vi "Initialize.vi"(8 "error in (no error)":errorcluster, 9 "Reset (True)":bool=TRUE, 10 "ID Query (True)":bool=TRUE, 11 "VISA resource name":refnum<visa-resource-name>) -> (0 "error out":errorcluster, 2 "idn string":string, 3 "VISA resource name out":refnum<visa-resource-name>, 5 "Model":u8(ring) items=["T3AWG3252", "T3AWG3352", "T3AWG3254", "T3AWG3354", "T3AWG3258", "T3AWG3358", "AWG4012", "AWG4014", "AWG4018", "Model675_2C", "Model675_4C", "Model675_8C", "Not valid"], 6 "Number of Markers Out":u8(ring) items=["1 Marker Out ", "2 Marker Out", "4 Marker Out"], 7 "Number of Channels Out":u8(ring) items=["2 Channels", "4 Channels", "8 Channels"])   [LabVIEW 2020, in "Active Technologies AWG3000.lvlib"]
doc: "Establishes communication with the instrument and optionally performs an instrument identification query and/or an instrument reset. It also places the instrument in a default state needed for other instrument driver operations. Therefore, call this VI before calling other instrument driver VIs for this instrument. Generally, you need to call the <B>Initialize VI</B> only once at the beginning of an application."
uses:
  Active Technologies AWG3000.lvlib
panel:
  in  "Timeout Value":u32=300000
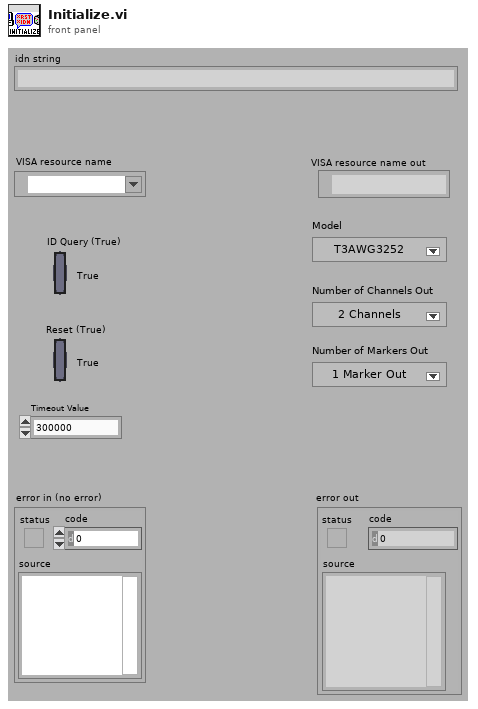
[diagram p1: front panel]
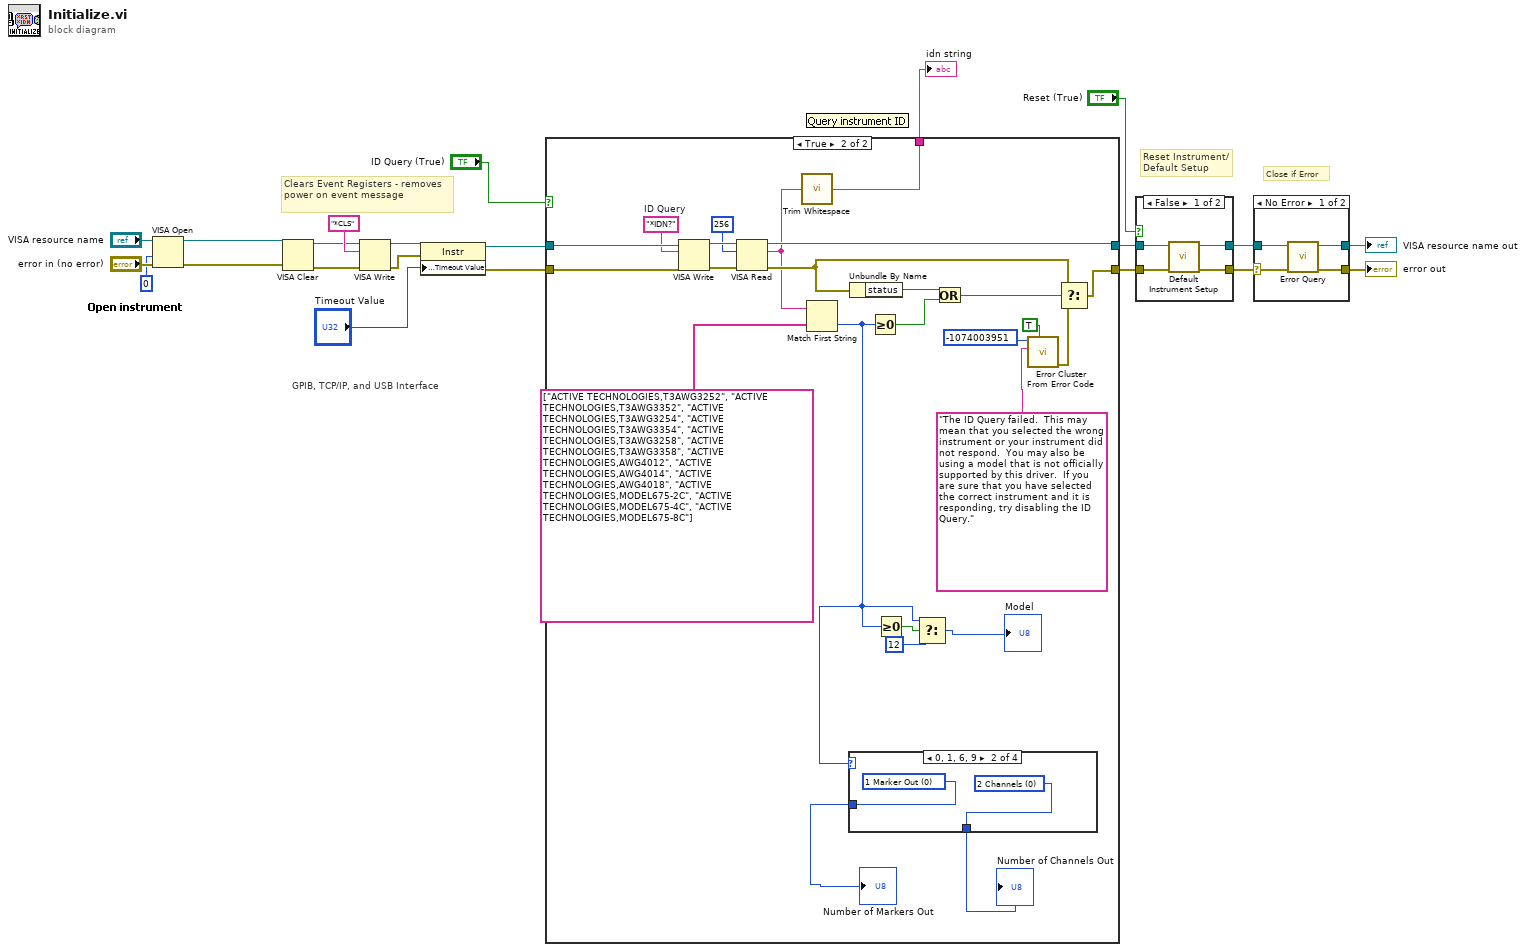
[diagram p0: block diagram]
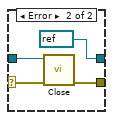
[diagram p2: hidden frame]
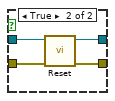
[diagram p3: hidden frame]
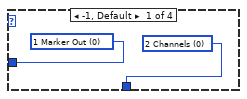
[diagram p5: hidden frame]
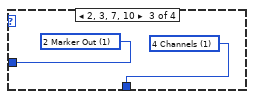
[diagram p6: hidden frame]
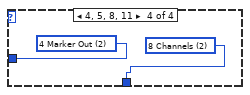
[diagram p7: hidden frame]
diagram:
  # "Clears Event Registers - removes power on event message"
  # "GPIB, TCP/IP, and USB Interface"
  # "Close if Error"
  # "Reset Instrument/\nDefault Setup"
  n1 = VISA Open(access mode=u32 0, error in (no error)="error in (no error)", VISA resource name="VISA resource name") -> (VISA resource name=w17:refnum<visa-resource-name>, error out=w16:errorcluster)  [unwired: 2 in]
  n2 = VISA Clear(VISA resource name=w17, error in (no error)=w16) -> (VISA resource name out=w5:refnum<visa-resource-name>, error out=w4:errorcluster)
  n3 = VISA Write(VISA resource name=w5, write buffer="*CLS", error in (no error)=w4) -> (VISA resource name out=w3:refnum<visa-resource-name>, error out=w2:errorcluster)  [unwired: 1 out]
  n4 = property class="Instr"(reference=w3, error in=w2, "General Settings:Timeout Value"="Timeout Value") -> (reference out=w9:refnum<visa-resource-name>, error out=w8:errorcluster)
  n5 = case shown="True" "ID Query (True)" {
    tunnel: [w23 w38] -> w10
    tunnel: [w24 w47] -> w11
    tunnel: w9 -> [w24 w48]
    tunnel: w8 -> [w23 w49]
    tunnel: [_ w25] -> w1
    frame False {
    }
    frame True {
      w43 = "*IDN?"  # ID Query
      n6 = VISA Write(VISA resource name=w48, write buffer=w43, error in (no error)=w49) -> (VISA resource name out=w46:refnum<visa-resource-name>, error out=w45:errorcluster)  [unwired: 1 out]
      n7 = VISA Read(VISA resource name=w46, byte count=u32 256, error in (no error)=w45) -> (VISA resource name out=w47:refnum<visa-resource-name>, read buffer=w26:string, error out=w42:errorcluster)  [unwired: 1 out]
      n8 = call <vilib>:"Trim Whitespace.vi"("string"=w26) -> ("trimmed string"=w25:string)  [unwired: 1 in]
      n9 = Match First String(2:string[] ["ACTIVE TECHNOLOGIES,T3AWG3252", "ACTIVE TECHNOLOGIES,T3AWG3352", "ACTIVE TECHNOLOGIES,T3AWG3254", "ACTIVE TECHNOLOGIES,T3AWG3354", "ACTIVE TECHNOLOGIES,T3AWG3258", "ACTIVE TECHNOLOGIES,T3AWG3358", "ACTIVE TECHNOLOGIES,AWG4012", "ACTIVE TECHNOLOGIES,AWG4014", "ACTIVE TECHNOLOGIES,AWG4018", "ACTIVE TECHNOLOGIES,MODEL675-2C", "ACTIVE TECHNOLOGIES,MODEL675-4C", "ACTIVE TECHNOLOGIES,MODEL675-8C"] ("reversed array"), 3:w26) -> (0:w30:i32)  [unwired: 1 out]
      n10 = case shown="0, 1, 6, 9" w30 {
        tunnel: [w51 w53 w55 w57] -> w33
        tunnel: [w50 w52 w54 w56] -> w32
        frame -1, Default {
          w50 = u8 0 items=["2 Channels", "4 Channels", "8 Channels"] ("Number of Channel Out")
          w51 = u8 0 items=["1 Marker Out ", "2 Marker Out", "4 Marker Out"] ("Number of Marker Out")
        }
        frame 0, 1, 6, 9 {
          w52 = u8 0 items=["2 Channels", "4 Channels", "8 Channels"] ("Number of Channel Out")
          w53 = u8 0 items=["1 Marker Out ", "2 Marker Out", "4 Marker Out"] ("Number of Marker Out")
        }
        frame 2, 3, 7, 10 {
          w54 = u8 1 items=["2 Channels", "4 Channels", "8 Channels"] ("Number of Channel Out")
          w55 = u8 1 items=["1 Marker Out ", "2 Marker Out", "4 Marker Out"] ("Number of Marker Out")
        }
        frame 4, 5, 8, 11 {
          w56 = u8 2 items=["2 Channels", "4 Channels", "8 Channels"] ("Number of Channel Out")
          w57 = u8 2 items=["1 Marker Out ", "2 Marker Out", "4 Marker Out"] ("Number of Marker Out")
        }
      }
      "Number of Markers Out" <- w33
      "Number of Channels Out" <- w32
      n11 = Unbundle By Name(w42) -> ("status"=w41:bool)
      n12 = Greater Or Equal To 0?(x=w30) -> (x >= 0?=w40:bool)
      n13 = Greater Or Equal To 0?(x=w30) -> (x >= 0?=w31:bool)
      n14 = Select(t=w30, s=w31, f=12) -> (s? t:f=→"Model":i32)
      n15 = Or(x=w41, y=w40) -> (x .or. y?=w39:bool)
      n16 = call <vilib>:"Error Cluster From Error Code.vi"("show call chain? (False)"=TRUE, "error message (\"\")"="The ID Query failed.  This may mean that you selected the wrong instrument or your instrument did not respond.  You may also be using a model that is not officially supported by this driver.  If you are sure that you have selected the correct instrument and it is responding, try disabling the ID Query." ("Source (VI Name)"), "error code (0)"=-1074003951 ("Code")) -> ("error out"=w34:errorcluster)  [unwired: 6 in]
      n17 = Select(t=w42, s=w39, f=w34) -> (s? t:f=w38:errorcluster)
    }
  }
  "idn string" <- w1
  n18 = case shown="False" "Reset (True)" {
    tunnel: [w60 w65] -> w12
    tunnel: w11 -> [w61 w63]
    tunnel: [w59 w64] -> w13
    tunnel: w10 -> [w58 w62]
    frame False {
      n19 = call "Default Instrument Setup.vi"("error in (no error)"=w58, "VISA resource name"=w61) -> ("error out"=w60:errorcluster, "VISA resource name out"=w59:refnum<visa-resource-name>)  [unwired: 8 in]
    }
    frame True {
      n20 = call "Reset.vi"("error in (no error)"=w62, "VISA resource name"=w63) -> ("error out"=w65:errorcluster, "VISA resource name out"=w64:refnum<visa-resource-name>)  [unwired: 8 in]
    }
  }
  n21 = case shown="No Error" w12 {
    selector: w12 -> [w67 w71]
    tunnel: w13 -> [w66 w72]
    tunnel: [w69 refnum<visa-resource-name> refnum ("VISA resource name out")] -> w15
    tunnel: [w68 w73] -> w14
    frame No Error {
      n22 = call "Error Query.vi"("error in (no error)"=w67, "VISA resource name"=w66) -> ("error out"=w68:errorcluster, "VISA resource name out"=w69:refnum<visa-resource-name>)  [unwired: 6 in, 2 out]
    }
    frame Error {
      n23 = call "Close.vi"("error in (no error)"=w71, "VISA resource name"=w72) -> ("error out"=w73:errorcluster)  [unwired: 9 in]
    }
  }
  "VISA resource name out" <- w15
  "error out" <- w14
